vi "SV Aures Sharpness (Time_2014) (1 Ch).vi"(0 "sound pressure signal [Pa]":waveform(dbl)={"t0"=timestamp(0 s since 1904-01-01), "dt"=1.953125e-05, "Y"=[]}, 1 "diffuse field":bool, 11 "error in (no error)":errorcluster) -> (4 "specific sharpness":T2, 6 "sharpness [acum]":dbl format="%.2f", 10 "sharpness info":T1, 15 "error out":errorcluster)   [LabVIEW 2017, in "SoundVib_SoundQuality.lvlib"]
doc: "Computes sharpness from the sound pressure signal waveform, the 1/3-octave band spectrum calculated over the frequency range 25 Hz to 12.5 kHz, or the specific loudness that the SV Stationary Loudness VI returns. Wire data to the <B>sound pressure signal [Pa]</B> input to determine the polymorphic instance to use or manually select the instance."
uses:
  <vilib>/addons/Sound and Vibration/svt_Sound Quality/SoundVib_SoundQuality.lvlib
  <vilib>/addons/_NISVFA/_Shared subVIs/Controls/svc_SQ Info.ctl
  <vilib>/addons/_NISVFA/_Shared subVIs/Common/SVL Set dB Reference (1 Ch).vi
  <vilib>/addons/_NISVFA/_Shared subVIs/Common/SVL Set dB Reference (variant).vi
  <vilib>/addons/Sound and Vibration/svt_Octave_2014 standard/SVT Third-octave Analysis (1 Ch).vi
  <vilib>/addons/_NISVFA/_Shared subVIs/Common/svc_Caller VI Returned in Error Source.vi
  <vilib>/addons/Sound and Vibration/svt_Octave/SoundVib_Octave_2014 standard.lvlib
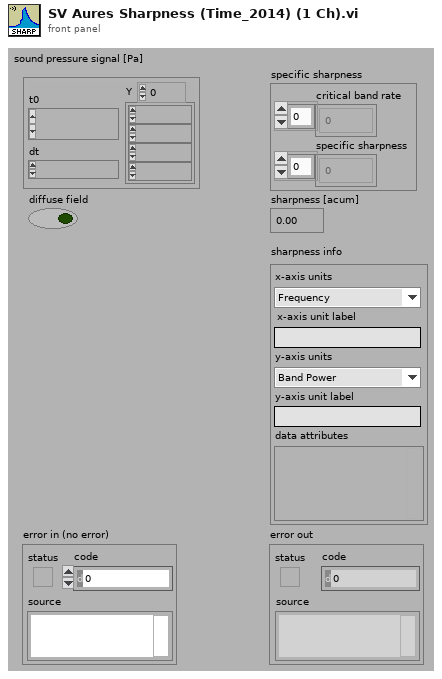
[diagram p1: front panel]
types:
  T1 = typedef "svc_SQ Info.ctl" = cluster{"x-axis units":enum16{"Frequency", "Critical Band", "Critical Band Rate"}, "x-axis unit label":string, "y-axis units":enum16{"Band Power", "Level", "Loudness", "Sharpness", "Roughness", "Fluctuation Strength", "Tonality"}, "y-axis unit label":string, "data attributes":variant}
  T2 = cluster{"critical band rate":dbl[], "specific sharpness":dbl[]}
  T3 = enum16{"Linear", "Exponential", "Equal confidence", "Peak"}
  T4 = cluster{"low band":enum16{"20 Hz", "25 Hz", "31.5 Hz", "40 Hz", "50 Hz", "63 Hz", "80 Hz", "100 Hz", "125 Hz", "160 Hz", "200 Hz", "250 Hz", "315 Hz", "400 Hz", "500 Hz", "630 Hz", "800 Hz", "1000 Hz", "1250 Hz", "1600 Hz", "2000 Hz", "2500 Hz", "3150 Hz", "4000 Hz", "5000 Hz", "6300 Hz", "8000 Hz", "10000 Hz", "12500 Hz", "16000 Hz", "20000 Hz"}, "high band":enum16{"20 Hz", "25 Hz", "31.5 Hz", "40 Hz", "50 Hz", "63 Hz", "80 Hz", "100 Hz", "125 Hz", "160 Hz", "200 Hz", "250 Hz", "315 Hz", "400 Hz", "500 Hz", "630 Hz", "800 Hz", "1000 Hz", "1250 Hz", "1600 Hz", "2000 Hz", "2500 Hz", "3150 Hz", "4000 Hz", "5000 Hz", "6300 Hz", "8000 Hz", "10000 Hz", "12500 Hz", "16000 Hz", "20000 Hz"}}
  T5 = cluster{"nominal frequencies [Hz]":dbl[], "band power":dbl[]}
  T6 = typedef "svc_Octave Info.ctl" = cluster{"standard":T7, "bandwidth":enum16{"1 octave", "1/3 octave", "1/6 octave", "1/12 octave", "1/24 octave"}, "low band":i32, "high band":i32, "weighting filter":T8, "dB reference":dbl, "dB On":bool, "unit label":string, "channel name":string, "description":string, "engineering units":T9, "custom label":string, "spectrum type":enum16{"power", "magnitude"}, "spectral density":bool, "filters settled":bool}
  T7 = typedef "svc_Octave Standard.ctl" = enum16{"ANSI S1.11", "IEC 61260"}
  T8 = typedef "svc_Weighting Filter Text Ring.ctl" = u16
  T9 = typedef "svc_Engineering Units Text Ring.ctl" = u16
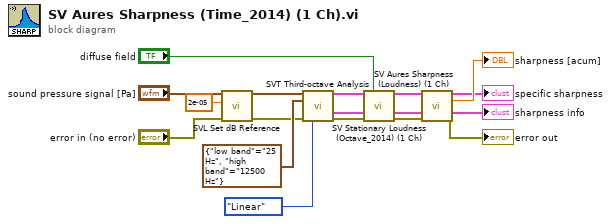
[diagram p0: block diagram]
diagram:
  n1 = call-poly <vilib>:"SVL Set dB Reference.vi"("error in (no error)"="error in (no error)", "dB reference [EU]"=2e-05, "scaled signal in [EU]"="sound pressure signal [Pa]") -> ("error out"=w2:errorcluster, "scaled signal out [EU]"=w4:waveform(dbl))  [unwired: 7 in]
  n2 = call-poly <vilib>:"SVT Third-octave Analysis.vi"("scaled signal [EU]"=w4, "frequency range"=T4 {"low band"=enum."25 Hz", "high band"=enum."12500 Hz"}, "error in (no error)"=w2, "averaging type"=T3."Linear") -> ("octave spectrum"=w7:T5, "octave info"=w8:T6, "error out"=w6:errorcluster)  [unwired: 6 in, 3 out]
  n3 = call <vilib>:"SV Stationary Loudness (Octave_2014) (1 Ch).vi"("octave spectrum"=w7, "diffuse field"="diffuse field", "octave info"=w8, "error in (no error)"=w6) -> ("specific loudness"=w15:cluster{dbl[], "Nm":dbl[]}, "loudness info"=w16:T1, "error out"=w17:errorcluster)  [unwired: 7 in, 2 out]
  n4 = call <vilib>:"SV Aures Sharpness (Loudness) (1 Ch).vi"("specific loudness"=w15, "loudness info"=w16, "error in (no error)"=w17) -> ("specific sharpness"=→"specific sharpness":T2, "sharpness [acum]"=→"sharpness [acum]":dbl, "sharpness info"=→"sharpness info":T1, "error out"=→"error out":errorcluster)  [unwired: 9 in]
